vi "GEA2 Serial Get ETX.vi"(8 "Error In":errorcluster, 10 "Current Read Index":i32, 11 "ReadArray":u8[](array[numeric])) -> (0 "Error Out":errorcluster, 2 "ETX = E3":bool, 3 "Current Read Index":i32)   [LabVIEW 2014]
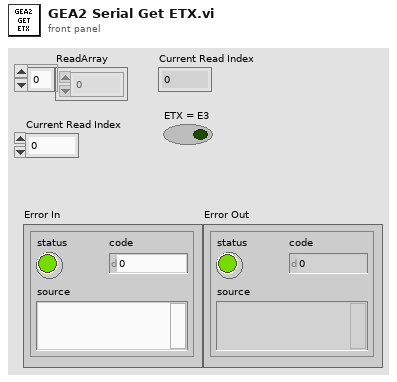
[diagram p1: front panel]
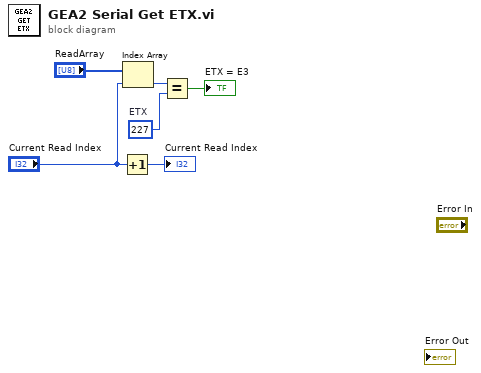
[diagram p0: block diagram]
diagram:
  w6 = u8 227  # ETX
  n1 = Increment(x="Current Read Index") -> (x+1=→"Current Read Index":i32)
  n2 = Index Array(array="ReadArray", index="Current Read Index") -> (element=w3:u8)
  n3 = Equal?(x=w3, y=w6) -> (x = y?=→"ETX = E3":bool)
